vi "_01_Sample_qsns_02[07].vi"() -> ()   [LabVIEW 2020]
panel:
  out "result string":string
  out "replaced substring":string
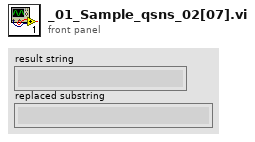
[diagram p1: front panel]
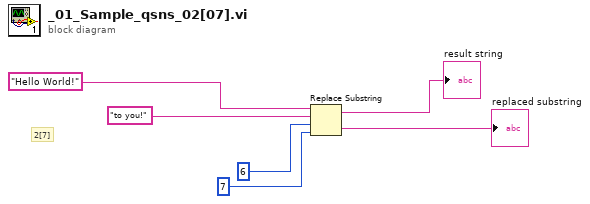
[diagram p0: block diagram]
diagram:
  # "2[7]"
  n1 = Replace Substring(2:7 ("length (len. of substring)"), 3:6 ("offset (0)"), 4:"to you!" ("substring (\"\")"), 5:"Hello World!" ("string")) -> (0:→"replaced substring":string, 1:→"result string":string)
